vi "RequestPulse.vi"(8 "error in (no error)":errorcluster, 11 "DMC 3600 in":refnum<class "DMC 3600.lvclass">) -> (0 "error out":errorcluster, 2 "Pulse":dbl, 3 "DMC 3600 out":refnum<class "DMC 3600.lvclass">)   [LabVIEW 2019, in "DMC 3600.lvclass"]
uses:
  DMC 3600.lvclass
  LLB/DMC3600/LTDMC.lvlib
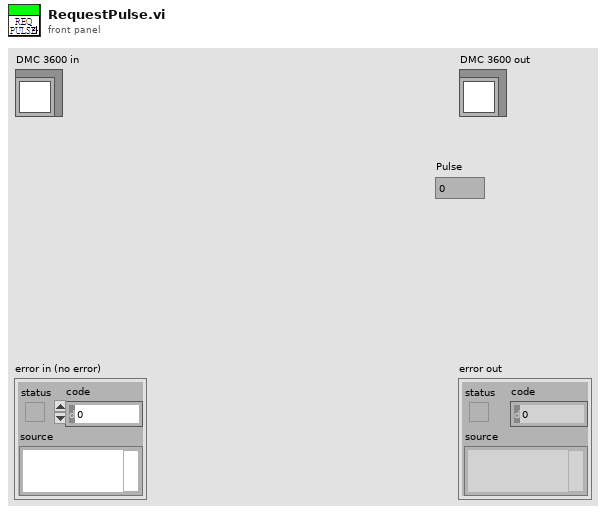
[diagram p1: front panel]
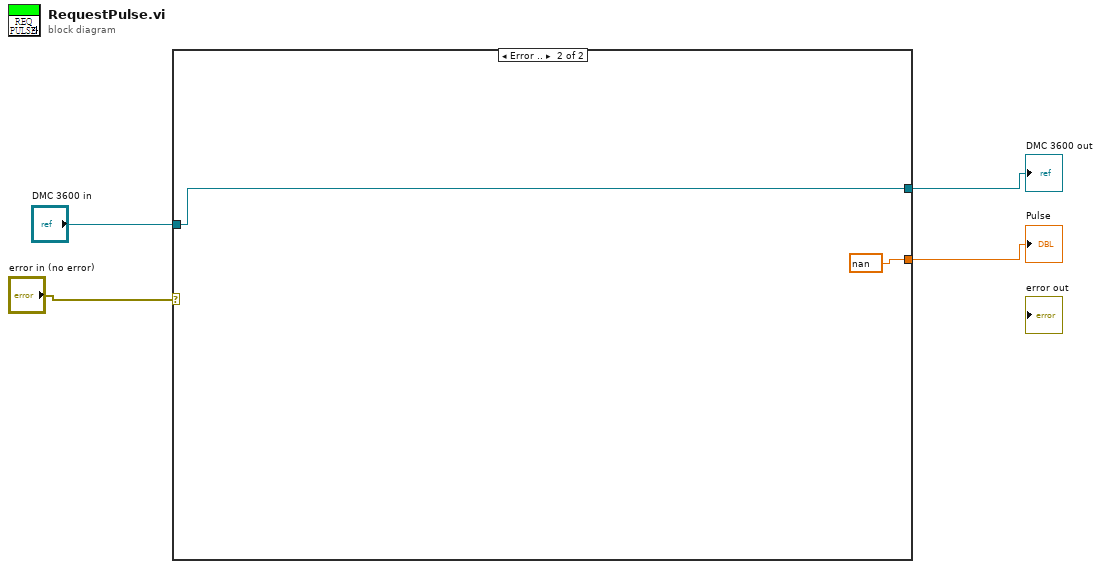
[diagram p0: block diagram]
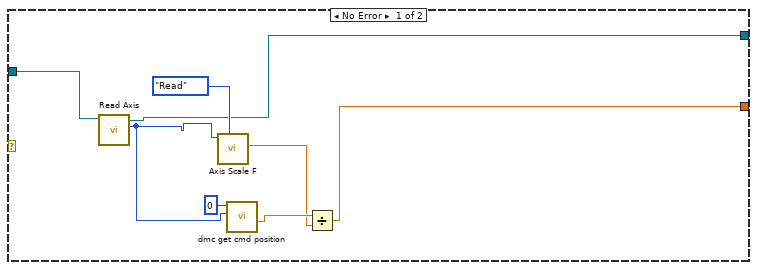
[diagram p2: hidden frame]
diagram:
  n1 = case shown="Error .." "error in (no error)" {
    tunnel: "DMC 3600 in" -> [w11 w14]
    tunnel: [w10 w14] -> w2
    tunnel: [w9 nan] -> w1
    frame No Error {
      n2 = call-dynamic "Read Axis.vi"("AxisCard in"=w11) -> ("Axis"=w7:u32, "AxisCard out"=w10:refnum<class "DMC 3600.lvclass">)  [unwired: 8 in, 1 out]
      n3 = call "Axis Scale F.vi"("Enum"=enum16{"Initial", "Read"}."Read", "Axis"=w7) -> ("Scale"=w5:dbl)  [unwired: 8 in, 1 out]
      n4 = call "dmc get cmd position.vi"("axis"=w7, "CardNo"=u16 0) -> ("pos out"=w6:dbl)  [unwired: 7 in, 2 out]
      n5 = Divide(x=w6, y=w5) -> (x/y=w9:dbl)
    }
    frame Error {
    }
  }
  "DMC 3600 out" <- w2
  "Pulse" <- w1
